vi "FindPreTriggerStart.vi"(8 "error in (no error)":errorcluster, 9 "data":T1, 10 "data event":T6, 11 "start block":T5) -> (0 "error out":errorcluster, 1 "not enough data":bool, 2 "start block out":T5, 3 "pretrigger start":T5)   [LabVIEW 2017, in "CmsDataEventCreator.lvlib"]
uses:
  <vilib>/addons/InsightCM/Devices/Shared/Cms/CmsDataEventCreator/CmsDataEventCreator.lvlib
  <vilib>/addons/InsightCM/Devices/Shared/Common/DVRBuffer/controls/BufferLocation.ctl
  <vilib>/addons/InsightCM/Devices/Shared/Cms/CmsDataEventCreator/controls/DataEventConfig.ctl
  <vilib>/addons/InsightCM/Devices/Shared/Cms/CmsDataEventCreator/controls/AcqParams.ctl
  <vilib>/addons/InsightCM/Devices/Shared/Common/DataAccumulator/controls/AccumulationSettings.ctl
  <vilib>/addons/InsightCM/Devices/Shared/Common/DataAccumulator/controls/accumulationType.ctl
  <vilib>/addons/PointValueMap/controls/PointMap.ctl
  <vilib>/addons/InsightCM/Devices/Shared/Common/DataFlow/controls/Data.ctl
  <vilib>/addons/InsightCM/Utilities/DataAccessors/controls/wfmSGL_DVR.ctl
  <vilib>/addons/InsightCM/Devices/Shared/Common/DataFlow/controls/Type.ctl
  <vilib>/addons/InsightCM/Devices/Shared/Common/DVRBuffer/DVRBuffer.lvlib
  <vilib>/addons/PointValueMap/PointValueMap.lvlib
  <vilib>/addons/InsightCM/Devices/Shared/Common/DataAccumulator/DataAccumulator.lvlib
  <vilib>/addons/InsightCM/Devices/Shared/Common/DataFlow/DataFlow.lvlib
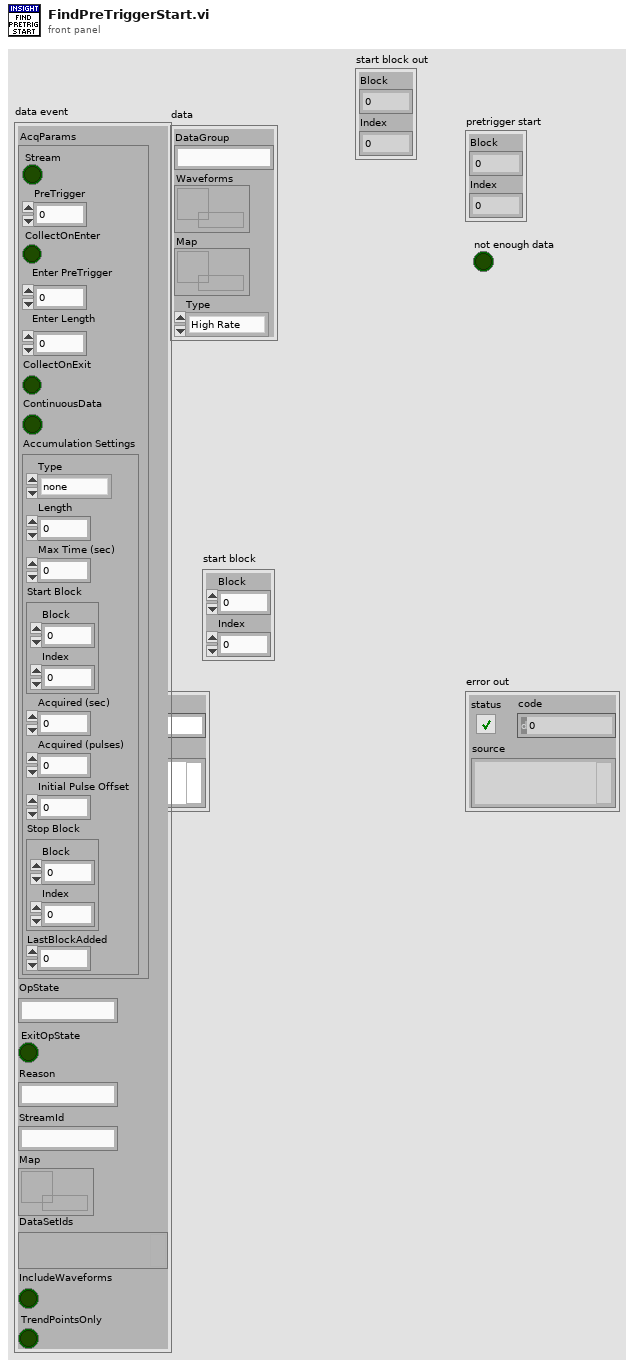
[diagram p1: front panel]
types:
  T1 = typedef "DataFlow.lvlib/Data.ctl" = cluster{"DataGroup":string, "Waveforms":T2, "Map":T3, "Type":T4}
  T2 = typedef "wfmSGL_DVR.ctl" = refnum<data-value>
  T3 = typedef "PointValueMap.lvlib/PointMap.ctl" = refnum<data-value>
  T4 = typedef "DataFlow.lvlib/Type.ctl" = enum16{"High Rate", "Low Rate", "Burst Mode"}
  T5 = typedef "DVRBuffer.lvlib/BufferLocation.ctl" = cluster{"Block":u32, "Index":i32}
  T6 = typedef "CmsDataEventCreator.lvlib/DataEventConfig.ctl" = cluster{"AcqParams":T7, "OpState":string, "ExitOpState":bool, "Reason":string, "StreamId":string, "Map":T3, "DataSetIds":variant, "IncludeWaveforms":bool, "TrendPointsOnly":bool}
  T7 = typedef "CmsDataEventCreator.lvlib/AcqParams.ctl" = cluster{"Stream":bool, "PreTrigger":i32, "CollectOnEnter":bool, "Enter PreTrigger":i32, "Enter Length":dbl, "CollectOnExit":bool, "ContinuousData":bool, "Accumulation Settings":T8}
  T8 = typedef "DataAccumulator.lvlib/AccumulationSettings.ctl" = cluster{"Type":T9, "Length":dbl, "Max Time (sec)":dbl, "Start Block":T5, "Acquired (sec)":dbl, "Acquired (pulses)":i32, "Initial Pulse Offset":dbl, "Stop Block":T5, "LastBlockAdded":u32}
  T9 = typedef "DataAccumulator.lvlib/accumulationType.ctl" = enum16{"none", "seconds", "revolutions"}
  T10 = typedef "DVRBuffer.lvlib/DVRElement.ctl" = cluster{"location":u32, "DVR":u32, "points":i32, "dt":dbl, "PulsePositions":dbl[], "Pulses Per Rev":dbl}
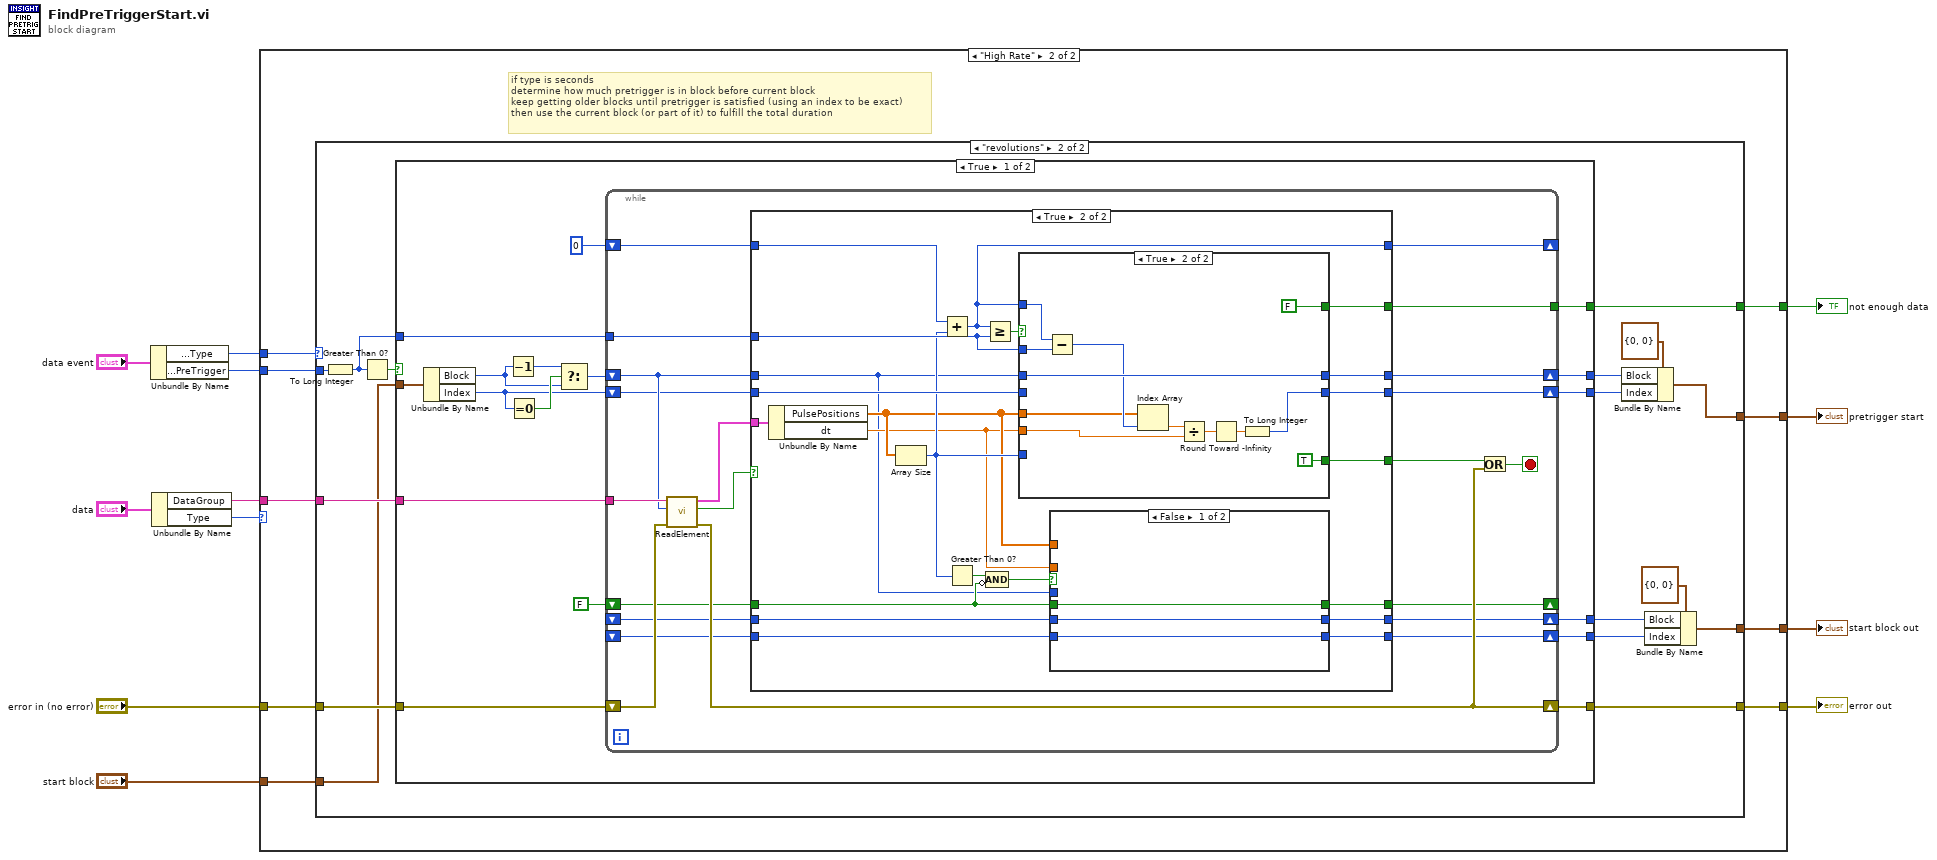
[diagram p0: block diagram]
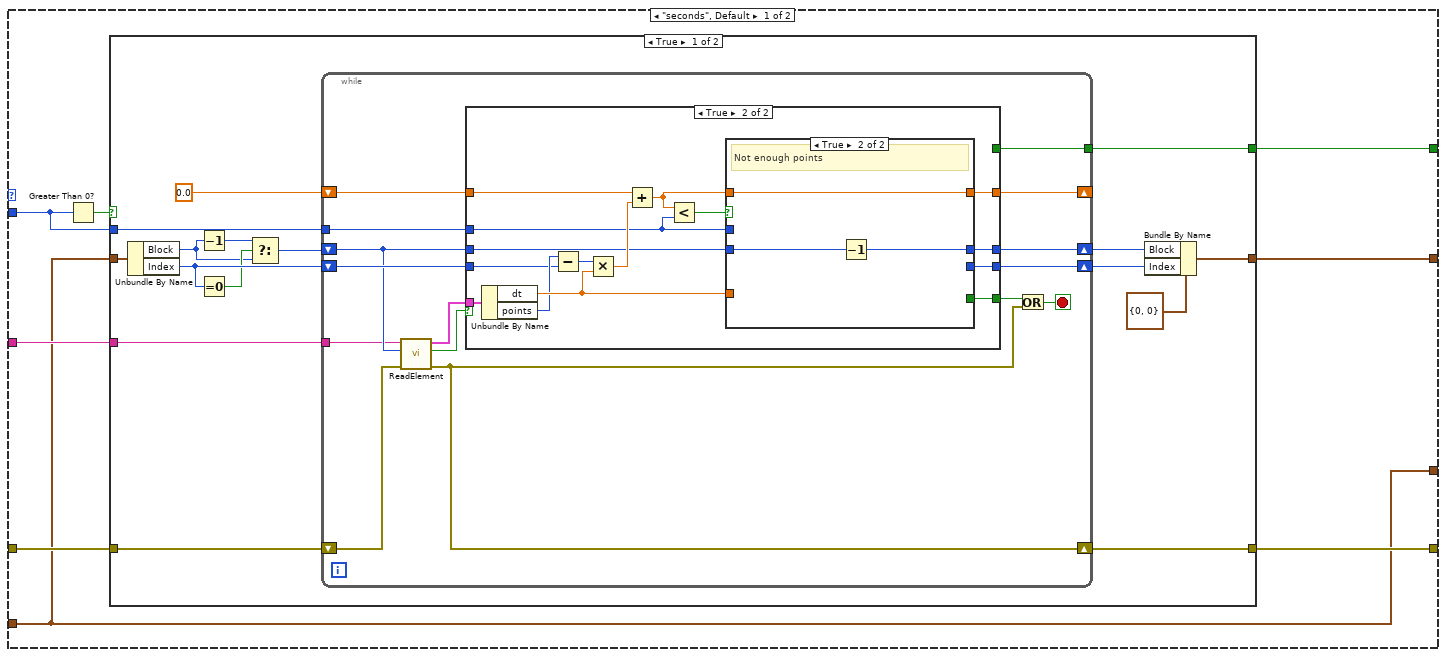
[diagram p3: hidden frame]
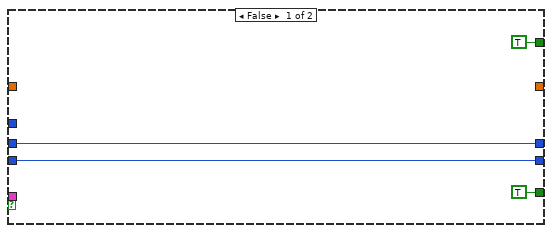
[diagram p4: hidden frame]
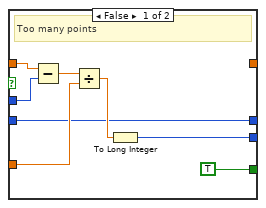
[diagram p5: hidden frame]
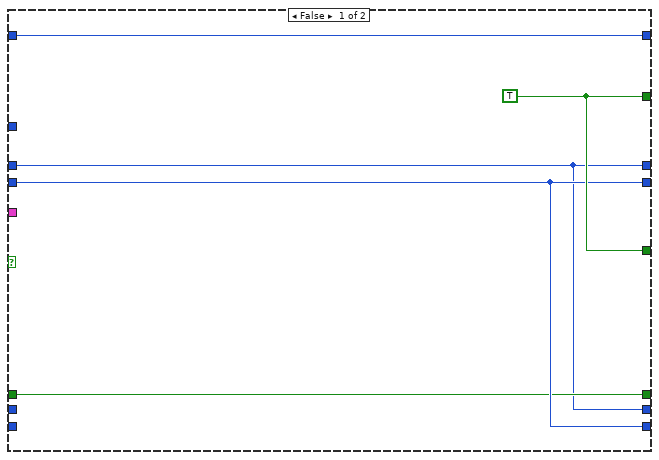
[diagram p7: hidden frame]
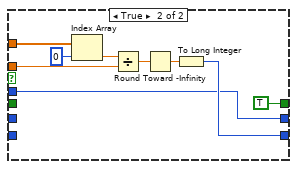
[diagram p8: hidden frame]
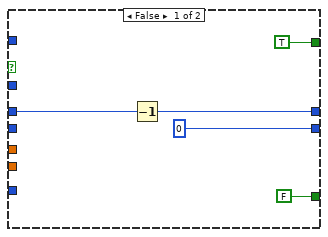
[diagram p9: hidden frame]
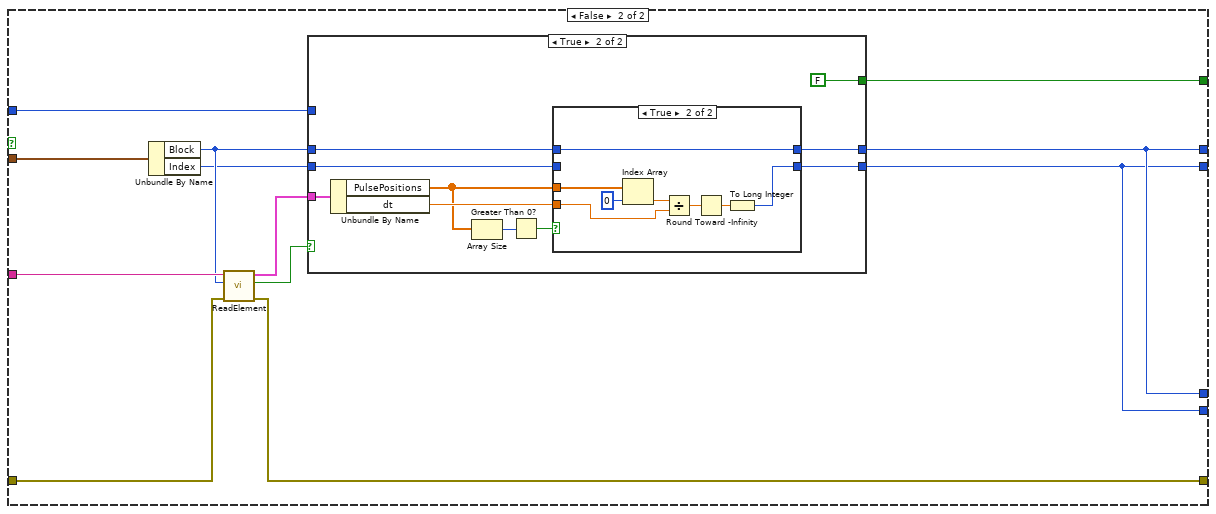
[diagram p10: hidden frame]
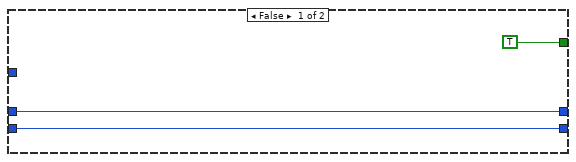
[diagram p11: hidden frame]
diagram:
  n1 = Unbundle By Name("data event") -> ("AcqParams.Accumulation Settings.Type"=w5:T9, "AcqParams.PreTrigger"=w6:i32)
  n2 = Unbundle By Name("data") -> ("DataGroup"=w3:string, "Type"=w1:T4)
  n3 = case shown="\"High Rate\"" w1 {
    tunnel: [_ w23] -> w12
    tunnel: [w13 w22] -> w11
    tunnel: "start block" -> [w14 w21]
    tunnel: "error in (no error)" -> [w13 w20]
    tunnel: [w14 w19] -> w8
    tunnel: w6 -> [_ w18]
    tunnel: w5 -> [_ w17]
    tunnel: [w14 w16] -> w4
    tunnel: w3 -> [_ w15]
    frame Default {
      # "If we are in the low rate data flow,\nignore pretrigger, just use the \nblock of data that we get from\nthe dataflow."
    }
    frame "High Rate" {
      # "if type is seconds\ndetermine how much pretrigger is in block before current block\nkeep getting older blocks until pretrigger is satisfied (using an index to be exact)\nthen use the current block (or part of it) to fulfill the total duration"
      n4 = case shown="\"revolutions\"" w17 {
        tunnel: [w31 w103] -> w23
        tunnel: [w30 w108] -> w22
        tunnel: w21 -> [w24 w99]
        tunnel: w20 -> [w29 w109]
        tunnel: [w28 w104] -> w19
        tunnel: w15 -> [w27 w110]
        tunnel: w18 -> [w26 w101]
        tunnel: [w24 w97] -> w16
        frame "seconds", Default {
          n5 = Greater Than 0?(x=w26) -> (x > 0?=w25:bool)
          n6 = case shown="True" w25 {
            tunnel: w26 -> [w47 _]
            tunnel: [w45 _] -> w31
            tunnel: [w44 w93] -> w30
            tunnel: w24 -> [w43 w94]
            tunnel: w29 -> [w42 w93]
            tunnel: [w38 w94] -> w28
            tunnel: w27 -> [w37 _]
            frame True {
              n7 = Unbundle By Name(w43) -> ("Block"=w32:u32, "Index"=w36:i32)
              n8 = Decrement(x=w32) -> (x-1=w34:u32)
              n9 = Equal To 0?(x=w36) -> (x = 0?=w35:bool)
              n10 = Select(t=w34, s=w35, f=w32) -> (s? t:f=w33:u32)
              n11 = while {
                tunnel: w47 -> [w61]
                shift-right: [w55] -> _
                shift-left: 0.0 -> [w60]
                shift-right: [w58] -> w39
                shift-left: w36 -> [w62]
                shift-right: [w57] -> w40
                shift-left: w33 -> [w59]
                tunnel: [w56] -> w45
                tunnel: w37 -> [w48]
                shift-right: [w52] -> w44
                shift-left: w42 -> [w49]
                stop <- w51 stop-if-true
                n12 = call <vilib>:"ReadElement.vi"("error in (no error)"=w49, "buffer location"=w59, "name"=w48) -> ("error out"=w52:errorcluster, "found"=w54:bool, "DVR element"=w53:T10)  [unwired: 6 in]
                n13 = case shown="True" w54 {
                  tunnel: w62 -> [w63 w68]
                  tunnel: w61 -> [_ w76]
                  tunnel: w60 -> [_ w81]
                  tunnel: w53 -> [_ w80]
                  tunnel: [TRUE w74] -> w50
                  tunnel: [w63 w73] -> w58
                  tunnel: [w64 w72] -> w57
                  tunnel: w59 -> [w64 w71]
                  tunnel: [TRUE _] -> w56
                  tunnel: [_ w70] -> w55
                  frame False {
                  }
                  frame True {
                    n14 = Unbundle By Name(w80) -> ("dt"=w75:dbl, "points"=w69:i32)
                    n15 = Subtract(x=w69, y=w68) -> (x-y=w67:i32)
                    n16 = Multiply(x=w67, y=w75) -> (x*y=w79:dbl)
                    n17 = Add(x=w81, y=w79) -> (x+y=w77:dbl)
                    n18 = Less?(x=w77, y=w76) -> (x < y?=w78:bool)
                    n19 = case shown="True" w78 {
                      tunnel: w77 -> [w89 w90]
                      tunnel: w76 -> [w88 _]
                      tunnel: w75 -> [w86 _]
                      tunnel: [TRUE _] -> w74
                      tunnel: [w82 _] -> w73
                      tunnel: [w83 w91] -> w72
                      tunnel: w71 -> [w83 w92]
                      tunnel: [_ w90] -> w70
                      frame False {
                        # "Too many points"
                        n20 = Subtract(x=w89, y=w88) -> (x-y=w87:dbl)
                        n21 = Divide(x=w87, y=w86) -> (x/y=w85:dbl)
                        n22 = To Long Integer(number=w85) -> (32bit integer=w82:i32)
                      }
                      frame True {
                        # "Not enough points"
                        n23 = Decrement(x=w92) -> (x-1=w91:u32)
                      }
                    }
                  }
                }
                n24 = Or(x=w50, y=w52) -> (x .or. y?=w51:bool)
              }
              n25 = Bundle By Name(cluster=T5 {"Block"=0, "Index"=0} ("buffer location"), "Block"=w40, "Index"=w39) -> (w38:T5)
            }
            frame False {
            }
          }
        }
        frame "revolutions" {
          n26 = To Long Integer(number=w101) -> (32bit integer=w100:i32)
          n27 = Greater Than 0?(x=w100) -> (x > 0?=w102:bool)
          n28 = case shown="True" w102 {
            tunnel: w110 -> [w127 w216]
            tunnel: w109 -> [w126 w215]
            tunnel: w99 -> [w125 w214]
            tunnel: [w124 w205] -> w108
            tunnel: [w123 w207] -> w106
            tunnel: [w122 w206] -> w105
            tunnel: [w121 w213] -> w103
            tunnel: w100 -> [w120 w212]
            tunnel: [w112 w207] -> w96
            tunnel: [w111 w206] -> w95
            frame True {
              n29 = Unbundle By Name(w125) -> ("Block"=w117:u32, "Index"=w115:i32)
              n30 = Decrement(x=w117) -> (x-1=w118:u32)
              n31 = Equal To 0?(x=w115) -> (x = 0?=w119:bool)
              n32 = Select(t=w118, s=w119, f=w117) -> (s? t:f=w116:u32)
              n33 = while {
                tunnel: w127 -> [w148]
                tunnel: w120 -> [w140]
                shift-right: [w139] -> w124
                shift-left: w126 -> [w147]
                shift-right: [w146] -> w123
                shift-left: w116 -> [w145]
                shift-right: [w144] -> w122
                shift-left: w115 -> [w143]
                tunnel: [w137] -> w121
                shift-right: [w134] -> _
                shift-left: 0 -> [w135]
                shift-right: [w130] -> w111
                shift-left: _ -> [w132]
                shift-right: [w131] -> _
                shift-left: FALSE -> [w133]
                shift-right: [w128] -> w112
                shift-left: _ -> [w129]
                stop <- w138 stop-if-true
                n34 = call <vilib>:"ReadElement.vi"("error in (no error)"=w147, "buffer location"=w145, "name"=w148) -> ("error out"=w139:errorcluster, "found"=w141:bool, "DVR element"=w142:T10)  [unwired: 6 in]
                n35 = case shown="True" w141 {
                  tunnel: w142 -> [_ w175]
                  tunnel: w145 -> [w149 w156]
                  tunnel: [w151 w174] -> w144
                  tunnel: [w149 w173] -> w146
                  tunnel: w143 -> [w151 w172]
                  tunnel: w140 -> [_ w170]
                  tunnel: [w153 w167] -> w137
                  tunnel: [w153 w168] -> w136
                  tunnel: w135 -> [w152 w169]
                  tunnel: [w152 w166] -> w134
                  tunnel: w133 -> [w150 w161]
                  tunnel: w132 -> [_ w159]
                  tunnel: [w150 w158] -> w131
                  tunnel: [w151 w157] -> w130
                  tunnel: w129 -> [_ w155]
                  tunnel: [w149 w154] -> w128
                  frame False {
                    w153 = TRUE
                  }
                  frame True {
                    n36 = Unbundle By Name(w175) -> ("PulsePositions"=w164:dbl[], "dt"=w163:dbl)
                    n37 = Array Size(array=w164) -> (size(s)=w165:i32)
                    n38 = Add(x=w169, y=w165) -> (x+y=w166:i32)
                    n39 = Greater Than 0?(x=w165) -> (x > 0?=w162:bool)
                    n40 = Greater Or Equal?(x=w166, y=w170) -> (x >= y?=w171:bool)
                    n41 = Compound Arithmetic op=AND(w162, invert w161) -> (w160:bool)
                    n42 = case shown="True" w171 {
                      tunnel: w163 -> [_ w193]
                      tunnel: [0 w203] -> w174
                      tunnel: w164 -> [_ w194]
                      tunnel: [w191 w202] -> w173
                      tunnel: w156 -> [w192 w202]
                      tunnel: w172 -> [_ _]
                      tunnel: w165 -> [_ _]
                      tunnel: w170 -> [_ w198]
                      tunnel: w166 -> [_ w199]
                      tunnel: [FALSE TRUE] -> w168
                      tunnel: [TRUE FALSE] -> w167
                      frame False {
                        n43 = Decrement(x=w192) -> (x-1=w191:u32)
                      }
                      frame True {
                        n44 = Subtract(x=w199, y=w198) -> (x-y=w195:i32)
                        n45 = Index Array(array=w194, index=w195) -> (element=w204:dbl)
                        n46 = Divide(x=w204, y=w193) -> (x/y=w201:dbl)
                        n47 = Round Toward -Infinity(1:w201) -> (0:w200:dbl)
                        n48 = To Long Integer(number=w200) -> (32bit integer=w203:i32)
                      }
                    }
                    n49 = case shown="False" w160 {
                      tunnel: w161 -> [w177 _]
                      tunnel: w164 -> [_ w183]
                      tunnel: w163 -> [_ w182]
                      tunnel: w159 -> [w178 _]
                      tunnel: [w177 TRUE] -> w158
                      tunnel: [w178 w180] -> w157
                      tunnel: w156 -> [_ w179]
                      tunnel: [w176 w179] -> w154
                      tunnel: w155 -> [w176 _]
                      frame False {
                      }
                      frame True {
                        n50 = Index Array(array=w183, index=0) -> (element=w186:dbl)
                        n51 = Divide(x=w186, y=w182) -> (x/y=w185:dbl)
                        n52 = Round Toward -Infinity(1:w185) -> (0:w184:dbl)
                        n53 = To Long Integer(number=w184) -> (32bit integer=w180:i32)
                      }
                    }
                  }
                }
                n54 = Or(x=w136, y=w139) -> (x .or. y?=w138:bool)
              }
            }
            frame False {
              n55 = Unbundle By Name(w214) -> ("Block"=w211:u32, "Index"=w210:i32)
              n56 = call <vilib>:"ReadElement.vi"("error in (no error)"=w215, "buffer location"=w211, "name"=w216) -> ("error out"=w205:errorcluster, "found"=w208:bool, "DVR element"=w209:T10)  [unwired: 6 in]
              n57 = case shown="True" w208 {
                tunnel: w209 -> [_ w229]
                tunnel: w211 -> [w219 w222]
                tunnel: [w218 w227] -> w206
                tunnel: [w219 w223] -> w207
                tunnel: w210 -> [w218 w221]
                tunnel: w212 -> [_ _]
                tunnel: [TRUE FALSE] -> w213
                frame False {
                }
                frame True {
                  n58 = Unbundle By Name(w229) -> ("PulsePositions"=w226:dbl[], "dt"=w228:dbl)
                  n59 = Array Size(array=w226) -> (size(s)=w225:i32)
                  n60 = Greater Than 0?(x=w225) -> (x > 0?=w224:bool)
                  n61 = case shown="True" w224 {
                    tunnel: w228 -> [_ w237]
                    tunnel: [w231 w236] -> w227
                    tunnel: w226 -> [_ w235]
                    tunnel: [w230 w234] -> w223
                    tunnel: w222 -> [w230 w234]
                    tunnel: w221 -> [w231 _]
                    frame False {
                    }
                    frame True {
                      n62 = Index Array(array=w235, index=0) -> (element=w238:dbl)
                      n63 = Divide(x=w238, y=w237) -> (x/y=w233:dbl)
                      n64 = Round Toward -Infinity(1:w233) -> (0:w232:dbl)
                      n65 = To Long Integer(number=w232) -> (32bit integer=w236:i32)
                    }
                  }
                }
              }
            }
          }
          n66 = Bundle By Name(cluster=T5 {"Block"=0, "Index"=0} ("start block"), "Block"=w106, "Index"=w105) -> (w104:T5)
          n67 = Bundle By Name(cluster=T5 {"Block"=0, "Index"=0} ("start block"), "Block"=w96, "Index"=w95) -> (w97:T5)
        }
      }
    }
  }
  "error out" <- w11
  "not enough data" <- w12
  "pretrigger start" <- w8
  "start block out" <- w4
